vi "Config.Gui.Run.vi"(8 "error in":errorcluster) -> (0 "error out":errorcluster, 3 "Ref":refnum<vi>)   [LabVIEW 2013]
uses:
  Tma.lib/string.llb/Join array to string.vi
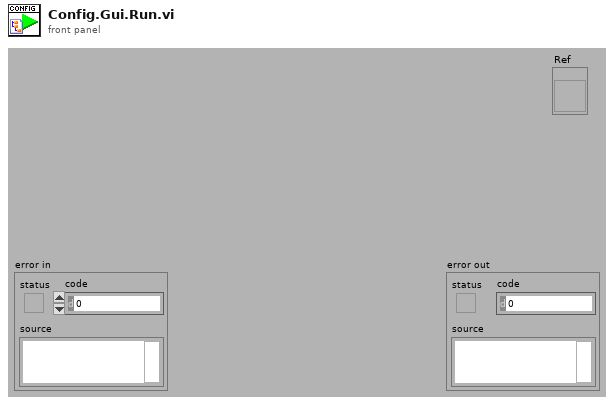
[diagram p1: front panel]
types:
  T1 = enum32{"Bad", "Idle", "Run top level", "Running"}
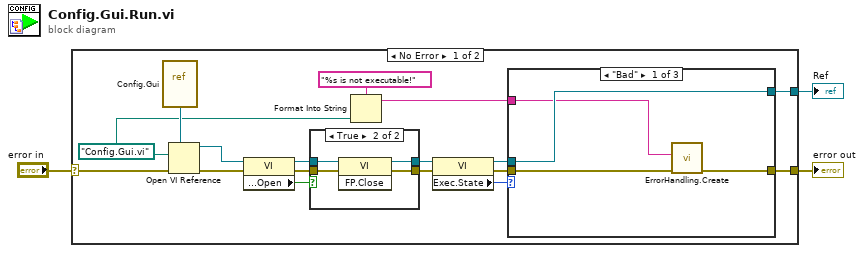
[diagram p0: block diagram]
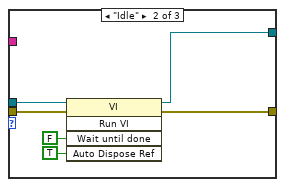
[diagram p3: hidden frame]
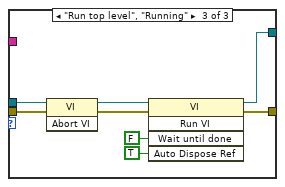
[diagram p4: hidden frame]
diagram:
  n1 = case shown="No Error" "error in" {
    selector: "error in" -> [w18 w45]
    tunnel: [w14 w45] -> w3
    tunnel: [w15 _] -> w1
    frame No Error {
      w5 = path "Config.Gui.vi" ("vi path")
      n2 = vi-ref "Config.Gui.vi"() -> (w19:refnum<vi>)
      n3 = Open VI Reference(type specifier VI Refnum (for type only)=w19, vi path=w5, error in (no error)=w18) -> (vi reference=w7:refnum<vi>, error out=w11:errorcluster)  [unwired: 3 in]
      n4 = property class="VI"(reference=w7, error in=w11) -> (reference out=w8:refnum<vi>, error out=w10:errorcluster, "Front Panel.Open"=w9:bool)
      n5 = case shown="True" w9 {
        tunnel: [w21 w26] -> w13
        tunnel: [w22 w25] -> w12
        tunnel: w10 -> [w21 w24]
        tunnel: w8 -> [w22 w23]
        frame False {
        }
        frame True {
          n6 = invoke class="VI" method="FP.Close"(reference=w23, error in=w24) -> (reference out=w25:refnum<vi>, error out=w26:errorcluster)  [unwired: 1 in, 1 out]
        }
      }
      n7 = Format Into String(format string="%s is not executable!" ("explanation"), w5) -> (resulting string=w4:string)  [unwired: 2 in, 1 out]
      n8 = property class="VI"(reference=w12, error in=w13) -> (reference out=w16:refnum<vi>, error out=w17:errorcluster, "Exec.State"=w20:T1)
      n9 = case shown="\"Bad\"" w20 {
        tunnel: [w28 w35 w38] -> w14
        tunnel: w17 -> [w29 w33 w42]
        tunnel: [w30 w34 w37] -> w15
        tunnel: w16 -> [w30 w36 w41]
        tunnel: w4 -> [w27 _ _]
        frame "Bad" {
          n10 = call "ErrorHandling.Create.vi"("error in"=w29, "explanation"=w27) -> ("error out"=w28:errorcluster)  [unwired: 9 in]
        }
        frame "Idle" {
          n11 = invoke class="VI" method="Run VI"(reference=w36, error in=w33, "Wait until done"=FALSE ("Wait Until Done"), "Auto Dispose Ref"=TRUE ("Auto Dispose Reference")) -> (reference out=w34:refnum<vi>, error out=w35:errorcluster)  [unwired: 1 in, 3 out]
        }
        frame "Run top level", "Running" {
          n12 = invoke class="VI" method="Abort VI"(reference=w41, error in=w42) -> (reference out=w39:refnum<vi>, error out=w40:errorcluster)  [unwired: 1 in, 1 out]
          n13 = invoke class="VI" method="Run VI"(reference=w39, error in=w40, "Wait until done"=FALSE ("Wait Until Done"), "Auto Dispose Ref"=TRUE ("Auto Dispose Reference")) -> (reference out=w37:refnum<vi>, error out=w38:errorcluster)  [unwired: 1 in, 3 out]
        }
      }
    }
    frame Error {
    }
  }
  "error out" <- w3
  "Ref" <- w1
